vi "Read Plugin Events.vi"(8 "error in (no error)":errorcluster, 11 "Session in":refnum<class "Plugin Session.lvclass">) -> (0 "error out":errorcluster, 2 "Plugin Events":T1, 3 "Session out":refnum<class "Plugin Session.lvclass">)   [LabVIEW 2021, in "CIF_InstrumentStudio Plugin SDK.lvlib" / "Plugin Session.lvclass"]
uses:
  Plugin Session.lvclass
  Plugin Events.ctl
  Plugin Session.lvclass/Plugin Session.ctl
  CIF_InstrumentStudio Plugin SDK.lvlib
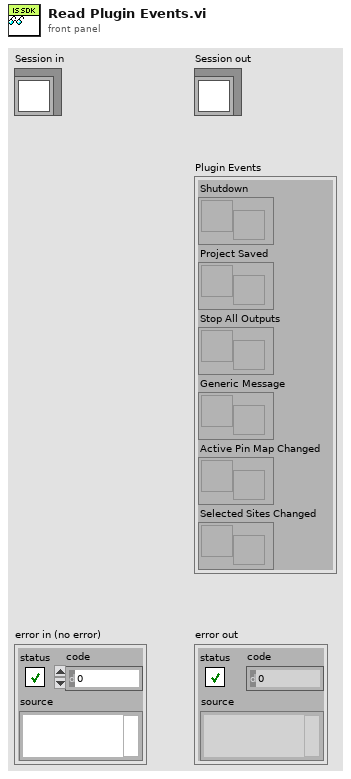
[diagram p1: front panel]
types:
  T1 = typedef "CIF_InstrumentStudio Plugin SDK.lvlib/Plugin Events.ctl" = cluster{"Shutdown":refnum<user-event>, "Project Saved":refnum<user-event>, "Stop All Outputs":refnum<user-event>, "Generic Message":refnum<user-event>, "Active Pin Map Changed":refnum<user-event>, "Selected Sites Changed":refnum<user-event>}
  T2 = typedef "InstrumentStudio Plugin SDK.lvlib/Plugin Events.ctl" = cluster{"Shutdown":refnum<user-event>, "Project Saved":refnum<user-event>, "Stop All Outputs":refnum<user-event>, "Generic Message":refnum<user-event>, "Active Pin Map Changed":refnum<user-event>, "Selected Sites Changed":refnum<user-event>}
  T3 = typedef "InstrumentStudio Plugin SDK.lvlib/Event Registration Refnum.ctl" = refnum<event-registration>
  T4 = cluster{"Session Id":u64, "Plugin Events":T2, "Event Refnum":T3}
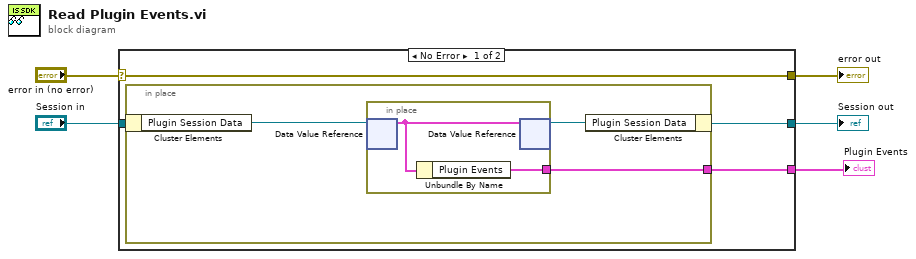
[diagram p0: block diagram]
diagram:
  n1 = case shown="No Error" "error in (no error)" {
    selector: "error in (no error)" -> [w9 w15]
    tunnel: [w9 w15] -> w4
    tunnel: [w6 w16] -> w2
    tunnel: "Session in" -> [w7 w16]
    tunnel: [w8 _] -> w1
    frame No Error {
      n2 = in-place {
        in-place-border: [w12] -> w8
        n3 = in-place-cluster #1(w7) -> ("Plugin Session Data"=w11:refnum<data-value>)
        n4 = in-place {
          in-place-border: [w14] -> w12
          n5 = in-place-dvr #2(w11) -> (w13:T4)  [unwired: 1 out]
          n6 = Unbundle By Name(w13) -> ("Plugin Events"=w14:T2)
          n7 = in-place-dvr #2(w13) -> (w10:refnum<data-value>)  [unwired: 1 out]
        }
        n8 = in-place-cluster #1("Plugin Session Data"=w10) -> (w6:refnum<class "Plugin Session.lvclass">)
      }
    }
    frame Error {
    }
  }
  "error out" <- w4
  "Session out" <- w2
  "Plugin Events" <- w1
